vi "Flower segement(SubVI).vi"(5 "Image in":T1, 6 "ROI 上半部分 2":T2={"Top"=0, "im_height"=1450, "L_left"=0, "im_width"=1680} caption="ROI 上半部分") -> (0 "黄色分量（油菜花）二值图":T1(plugin-control), 1 "黄色分量（油菜花）":T1(plugin-control), 2 "黄色分量（油菜花）Gray":T1(plugin-control), 3 "Number of Particles":i32, 4 "RGB花标记":T1(plugin-control))   [LabVIEW 2015]
uses:
  <vilib>/vision/Image Controls.llb/IMAQ Image.ctl
  <vilib>/vision/NI_Vision_Development_Module.lvlib
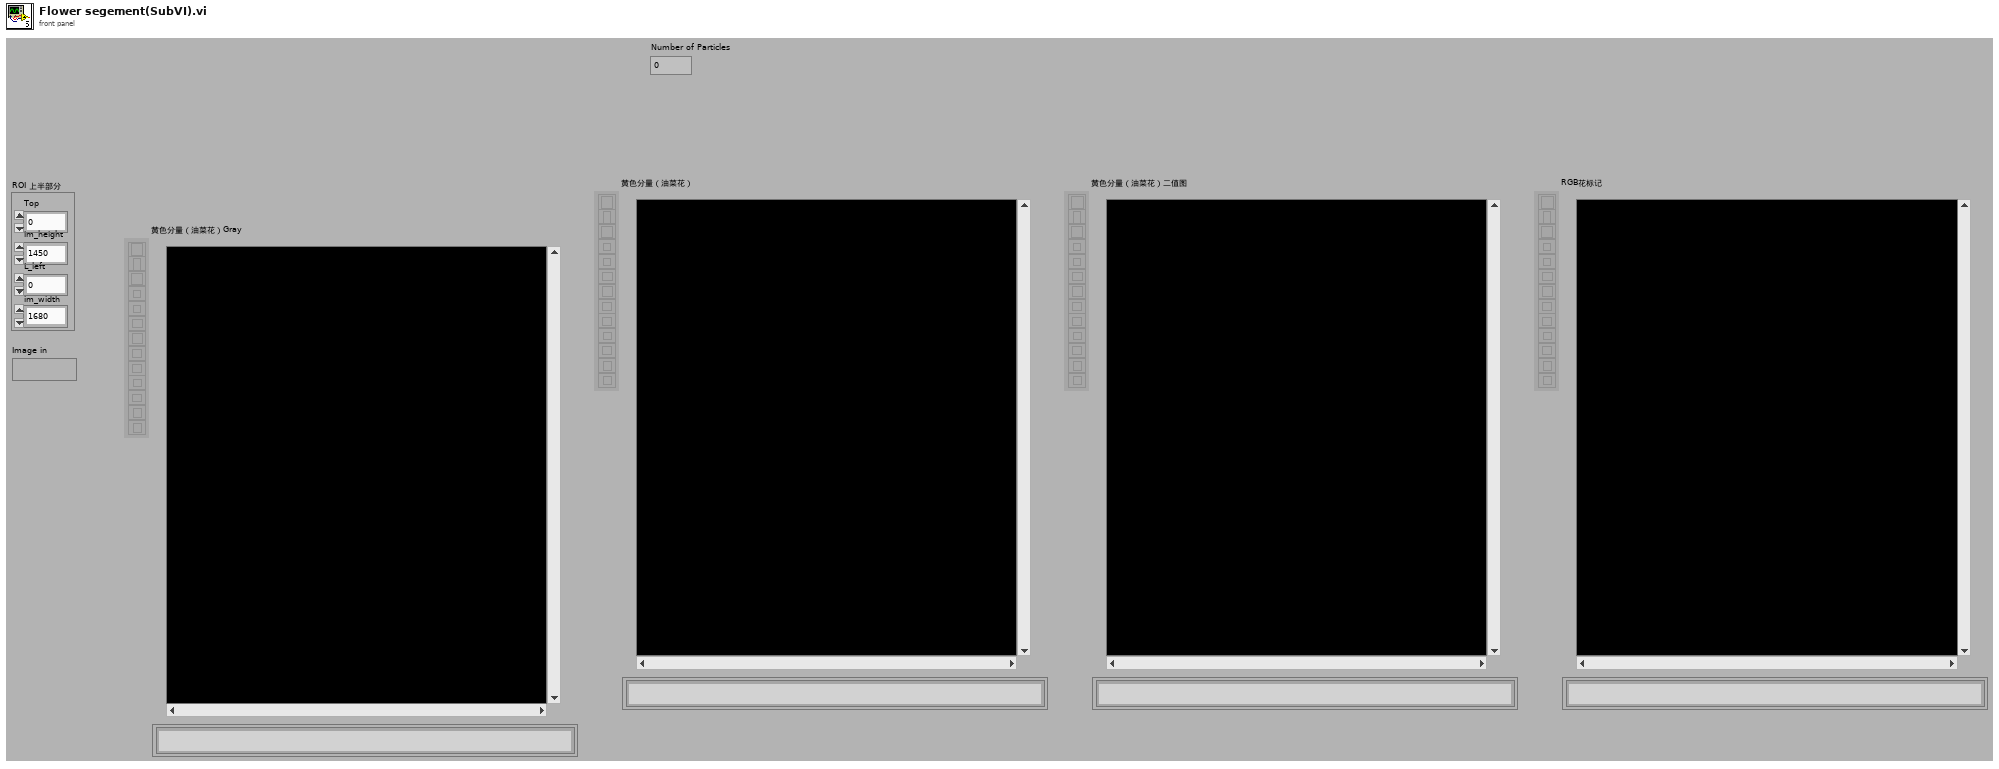
[diagram p1: front panel]
types:
  T1 = typedef "IMAQ Image.ctl" = refnum<image>
  T2 = cluster{"Top":i32, "im_height":i32, "L_left":i32, "im_width":i32}
  T3 = typedef "Image Type" = u32
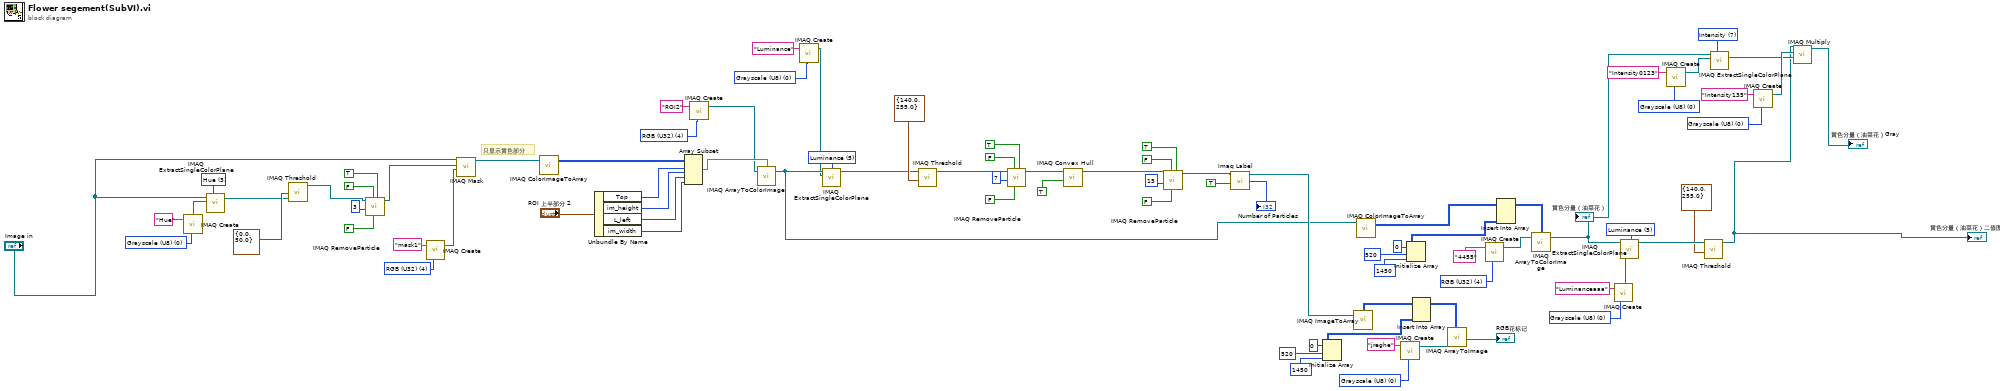
[diagram p0: block diagram]
diagram:
  w80 = T3 0 items=["Grayscale (U8)", "Grayscale (I16)", "Grayscale (SGL)", "Complex (CSG)", "RGB (U32)", "HSL (U32)", "RGB (U64)", "Grayscale (U16)"] ("Image Type")
  w83 = T3 0 items=["Grayscale (U8)", "Grayscale (I16)", "Grayscale (SGL)", "Complex (CSG)", "RGB (U32)", "HSL (U32)", "RGB (U64)", "Grayscale (U16)"] ("Image Type")
  w84 = 7 items=["Red", "Green", "Blue", "Hue", "Saturation", "Luminance", "Value", "Intensity"] ("Color Plane")
  w35 = u32 0 items=["Grayscale (U8)", "Grayscale (I16)", "Grayscale (SGL)", "Complex (CSG)", "RGB (U32)", "HSL (U32)", "RGB (U64)"] ("Image Type")
  w46 = 5 items=["Red", "Green", "Blue", "Hue", "Saturation", "Luminance", "Value", "Intensity"] ("Color Plane")
  w49 = u32 4 items=["Grayscale (U8)", "Grayscale (I16)", "Grayscale (SGL)", "Complex (CSG)", "RGB (U32)", "HSL (U32)", "RGB (U64)"] ("Image Type")
  w53 = u32 4 items=["Grayscale (U8)", "Grayscale (I16)", "Grayscale (SGL)", "Complex (CSG)", "RGB (U32)", "HSL (U32)", "RGB (U64)"] ("Image Type")
  w57 = u32 0 items=["Grayscale (U8)", "Grayscale (I16)", "Grayscale (SGL)", "Complex (CSG)", "RGB (U32)", "HSL (U32)", "RGB (U64)"] ("Image Type")
  w60 = 3 items=["Red", "Green", "Blue", "Hue", "Saturation", "Luminance", "Value", "Intensity"] ("Color Plane")
  w28 = u32 0 items=["Grayscale (U8)", "Grayscale (I16)", "Grayscale (SGL)", "Complex (CSG)", "RGB (U32)", "HSL (U32)", "RGB (U64)"] ("Image Type")
  w31 = 5 items=["Red", "Green", "Blue", "Hue", "Saturation", "Luminance", "Value", "Intensity"] ("Color Plane")
  w22 = u32 4 items=["Grayscale (U8)", "Grayscale (I16)", "Grayscale (SGL)", "Complex (CSG)", "RGB (U32)", "HSL (U32)", "RGB (U64)"] ("Image Type")
  w13 = u32 0 items=["Grayscale (U8)", "Grayscale (I16)", "Grayscale (SGL)", "Complex (CSG)", "RGB (U32)", "HSL (U32)", "RGB (U64)"] ("Image Type")
  # "只显示黄色部分"
  n1 = call "IMAQ Create"("Image Name"="Hue", "Image Type"=w57) -> ("New Image"=w56:T1)  [unwired: 2 in, 2 out]
  n2 = call "IMAQ ExtractSingleColorPlane"("Color Plane"=w60, "Image Dst"=w56, "Image Src"="Image in") -> ("Image Dst Out"=w58:T1)  [unwired: 1 in, 7 out]
  n3 = call "IMAQ Threshold"("Range"=cluster{"Lower value":sgl, "Upper value":sgl} {"Lower value"=0.0, "Upper value"=50.0}, "Image Src"=w58) -> ("Image Dst Out"=w3:T1)  [unwired: 4 in, 5 out]
  n4 = call "IMAQ RemoveParticle"("Connectivity 4/8 (8)"=TRUE, "Low Pass/High Pass (Low)"=FALSE, "Square/Hexa (Square)"=FALSE, "Number of Erosion"=3, "Image Src"=w3) -> ("Image Dst Out"=w2:T1)  [unwired: 2 in, 4 out]
  n5 = call "IMAQ Create"("Image Name"="mask1", "Image Type"=w53) -> ("New Image"=w52:T1)  [unwired: 2 in, 2 out]
  n6 = call "IMAQ Mask"("Image Dst"=w52, "Image Mask"=w2, "Image Src"="Image in") -> ("Image Dst Out"=w61:T1)  [unwired: 1 in, 2 out]
  n7 = call "IMAQ ColorImageToArray"("Image"=w61) -> ("Image Pixels (U32)"=w51:u32[][])  [unwired: 2 in, 3 out]
  n8 = Unbundle By Name("ROI 上半部分 2") -> ("Top"=w67:i32, "im_height"=w68:i32, "L_left"=w69:i32, "im_width"=w70:i32)
  n9 = Array Subset(array=w51, index (row)=w67, length (row)=w68, index (col)=w69, length (col)=w70) -> (w48:u32[][])
  n10 = call "IMAQ Create"("Image Name"="ROI2", "Image Type"=w49) -> ("New Image"=w47:T1)  [unwired: 2 in, 2 out]
  n11 = call "IMAQ ArrayToColorImage"("Image Pixels (U32)"=w48, "Image"=w47) -> ("Image Out"=w74:T1)  [unwired: 2 in, 2 out]
  n12 = call "IMAQ Create"("Image Name"="Luminance", "Image Type"=w35) -> ("New Image"=w34:T1)  [unwired: 2 in, 2 out]
  n13 = call "IMAQ ExtractSingleColorPlane"("Color Plane"=w46, "Image Dst"=w34, "Image Src"=w74) -> ("Image Dst Out"=w44:T1)  [unwired: 1 in, 7 out]
  n14 = call "IMAQ Threshold"("Range"=cluster{"Lower value":sgl, "Upper value":sgl} {"Lower value"=140.0, "Upper value"=255.0}, "Image Src"=w44) -> ("Image Dst Out"=w39:T1)  [unwired: 4 in, 5 out]
  n15 = call "IMAQ RemoveParticle"("Connectivity 4/8 (8)"=TRUE, "Low Pass/High Pass (Low)"=FALSE, "Square/Hexa (Square)"=FALSE, "Number of Erosion"=7, "Image Src"=w39) -> ("Image Dst Out"=w38:T1)  [unwired: 2 in, 4 out]
  n16 = call "IMAQ Convex Hull"("Connectivity 4/8 (8)"=TRUE, "Image Src"=w38) -> ("Image Dst Out"=w66:T1)  [unwired: 2 in, 7 out]
  n17 = call "IMAQ RemoveParticle"("Connectivity 4/8 (8)"=TRUE, "Low Pass/High Pass (Low)"=FALSE, "Square/Hexa (Square)"=FALSE, "Number of Erosion"=15, "Image Src"=w66) -> ("Image Dst Out"=w73:T1)  [unwired: 2 in, 4 out]
  n18 = call "Imaq Label"("Connectivity 4/8 (8)"=TRUE, "Image Src"=w73) -> ("Number of Particles"=→"Number of Particles":i32, "Image Dst Out"=w75:T1)  [unwired: 2 in, 1 out]
  n19 = Initialize Array(u8 0 ("element"), 520 ("dimension size"), 1450 ("dimension size")) -> (w16:u8[][])
  n20 = call "IMAQ ImageToArray"("Image"=w75) -> ("Image Pixels (U8)"=w17:u8[][])  [unwired: 2 in, 5 out]
  n21 = call "IMAQ ColorImageToArray"("Image"=w74) -> ("Image Pixels (U32)"=w24:u32[][])  [unwired: 2 in, 3 out]
  n22 = call "IMAQ Create"("Image Name"="jreghe", "Image Type"=w13) -> ("New Image"=w14:T1)  [unwired: 2 in, 2 out]
  n23 = Initialize Array(u8 0 ("element"), 520 ("dimension size"), 1450 ("dimension size")) -> (w23:u8[][])
  n24 = Insert Into Array(array=w17, new element=w16) -> (w15:u8[][])  [unwired: 2 in]
  n25 = call "IMAQ ArrayToImage"("Image Pixels (U8)"=w15, "Image"=w14) -> ("Image Out"=→"RGB花标记":T1)  [unwired: 4 in, 5 out]
  n26 = call "IMAQ Create"("Image Name"="4455", "Image Type"=w22) -> ("New Image"=w26:T1)  [unwired: 2 in, 2 out]
  n27 = Insert Into Array(array=w24, new element=w23) -> (w25:u32[][])  [unwired: 2 in]
  n28 = call "IMAQ ArrayToColorImage"("Image Pixels (U32)"=w25, "Image"=w26) -> ("Image Out"=w85:T1)  [unwired: 2 in, 2 out]
  "黄色分量（油菜花）" <- w85
  n29 = call "IMAQ Create"("Image Name"="Luminanceaaa", "Image Type"=w28) -> ("New Image"=w27:T1)  [unwired: 2 in, 2 out]
  n30 = call "IMAQ ExtractSingleColorPlane"("Color Plane"=w31, "Image Dst"=w27, "Image Src"=w85) -> ("Image Dst Out"=w76:T1)  [unwired: 1 in, 7 out]
  n31 = call "IMAQ Create"("Image Name"="Intensity0123", "Image Type"=w83) -> ("New Image"=w77:T1)  [unwired: 2 in, 2 out]
  n32 = call "IMAQ Threshold"("Range"=cluster{"Lower value":sgl, "Upper value":sgl} {"Lower value"=140.0, "Upper value"=255.0}, "Image Src"=w76) -> ("Image Dst Out"=w8:T1)  [unwired: 4 in, 5 out]
  "黄色分量（油菜花）二值图" <- w8
  n33 = call "IMAQ ExtractSingleColorPlane"("Color Plane"=w84, "Image Dst"=w77, "Image Src"=w85) -> ("Image Dst Out"=w78:T1)  [unwired: 1 in, 7 out]
  n34 = call "IMAQ Create"("Image Name"="Intensity135", "Image Type"=w80) -> ("New Image"=w79:T1)  [unwired: 2 in, 2 out]
  n35 = call "IMAQ Multiply"("Image Src A"=w8, "Image Dst"=w79, "Image Src B"=w78) -> ("Image Dst Out"=→"黄色分量（油菜花）Gray":T1)  [unwired: 2 in, 3 out]
